vi "Set Colour Key.vi"(8 "error in":errorcluster, 9 "Key":u32 format="%.0x", 10 "Flag":bool, 11 "Surface Pointer":u32 format="%.0x") -> (0 "error out":errorcluster, 3 "Return":i32)   [LabVIEW 2015, in "LibSDL2.lvlib"]
uses:
  LibSDL2.lvlib
  DLL/SDL2.dll
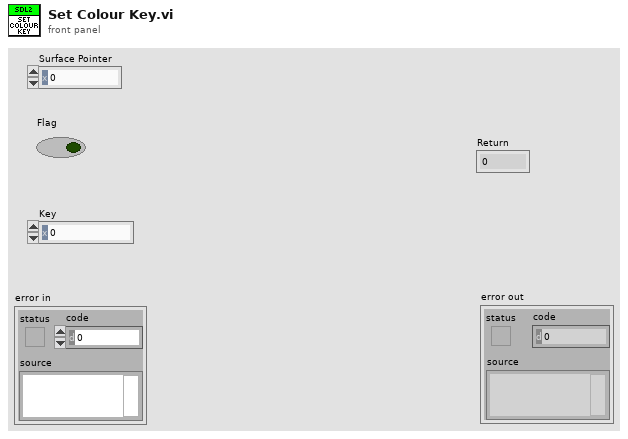
[diagram p1: front panel]
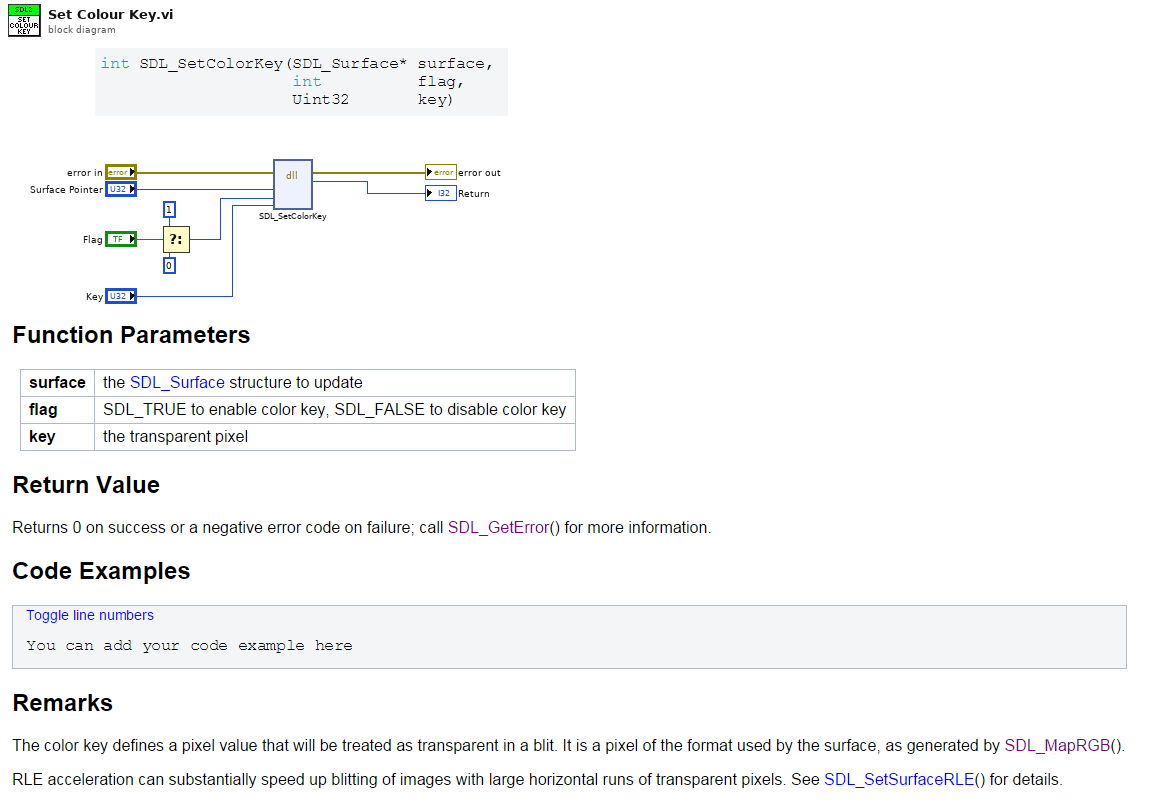
[diagram p0: block diagram]
diagram:
  n1 = Select(t=1, s="Flag", f=0) -> (s? t:f=w1:i32)
  n2 = dll-call lib="C:/dev/PGS/LabSDL2/Source/Libraries/LibSDL2 Wrapper/DLL/SDL2.dll" fn="SDL_SetColorKey"(error in="error in", "surface"="Surface Pointer", "flag"=w1, "key"="Key") -> (error out=→"error out":errorcluster, "return type"=→"Return":i32)  [unwired: 5 in, 1 out]
